vi "Read Config File.vi"(0 "file path":path=path "/home/lvuser/_config.ini", 1 "key":string) -> (2 "value":dbl, 3 "found?":bool, 4 "file path":path=path "/home/lvuser/_config.ini")   [LabVIEW 2014]
uses:
  <vilib>/Utility/config.llb/Read Key (Double).vi
  <vilib>/Utility/config.llb/NI_LVConfig.lvlib
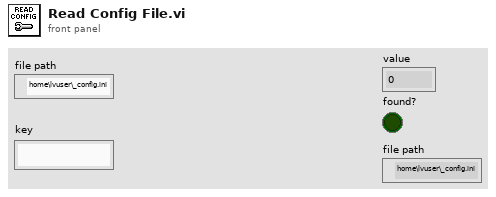
[diagram p1: front panel]
types:
  T1 = typedef "NI_LVConfig.lvlib/Config Data RefNum.ctl" = refnum<k1>
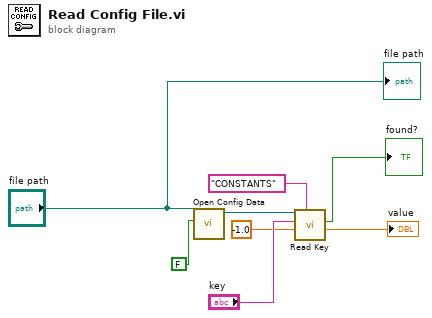
[diagram p0: block diagram]
diagram:
  n1 = call <vilib>:"Open Config Data.vi"("create file if necessary (T)"=FALSE, "configuration file path"="file path") -> ("refnum"=w7:T1)  [unwired: 7 in, 2 out]
  n2 = call-poly <vilib>:"Read Key.vi"("section"="CONSTANTS", "default value"=-1.0, "key"="key", "refnum"=w7) -> ("value"=→"value":dbl, "found?"=→"found?":bool)  [unwired: 4 in, 2 out]
  "file path" <- "file path"
